vi "PCO_GetCameraDescription.vi"(8 "error in (no error)":errorcluster {"code" format="%x"}, 11 "ph":u64) -> (0 "error out":errorcluster {"code" format="%x"}, 1 "strDescription":T1 {"wSensorTypeDESC" format="%x"; "wSensorSubTypeDESC" format="%x"; "wColorPatternDESC" format="%x"; "wPatternTypeDESC" format="%x"; "dwGeneralCapsDESC1" format="%x"; "dwGeneralCapsDESC2" format="%x"; "dwGeneralCapsDESC3" format="%x"; "dwGeneralCapsDESC4" format="%x"}, 2 "ErrorMessage":i32 format="%x", 3 "ph out":u64)   [LabVIEW 2020, in "SDK.lvlib" / "CameraDescription.lvlib"]
doc: "<b>Description:</b>\nSensor and camera specific description is queried. In the returned PCO_Description structure margins for all sensor related settings and bitfields for available options of the camera are given.\n\n<b>Supported camera type:</b>\nAll cameras\n\n<b>Descriptor dependency:</b>\nNone"
uses:
  CameraDescription.lvlib
  Structures/Structures.lvlib
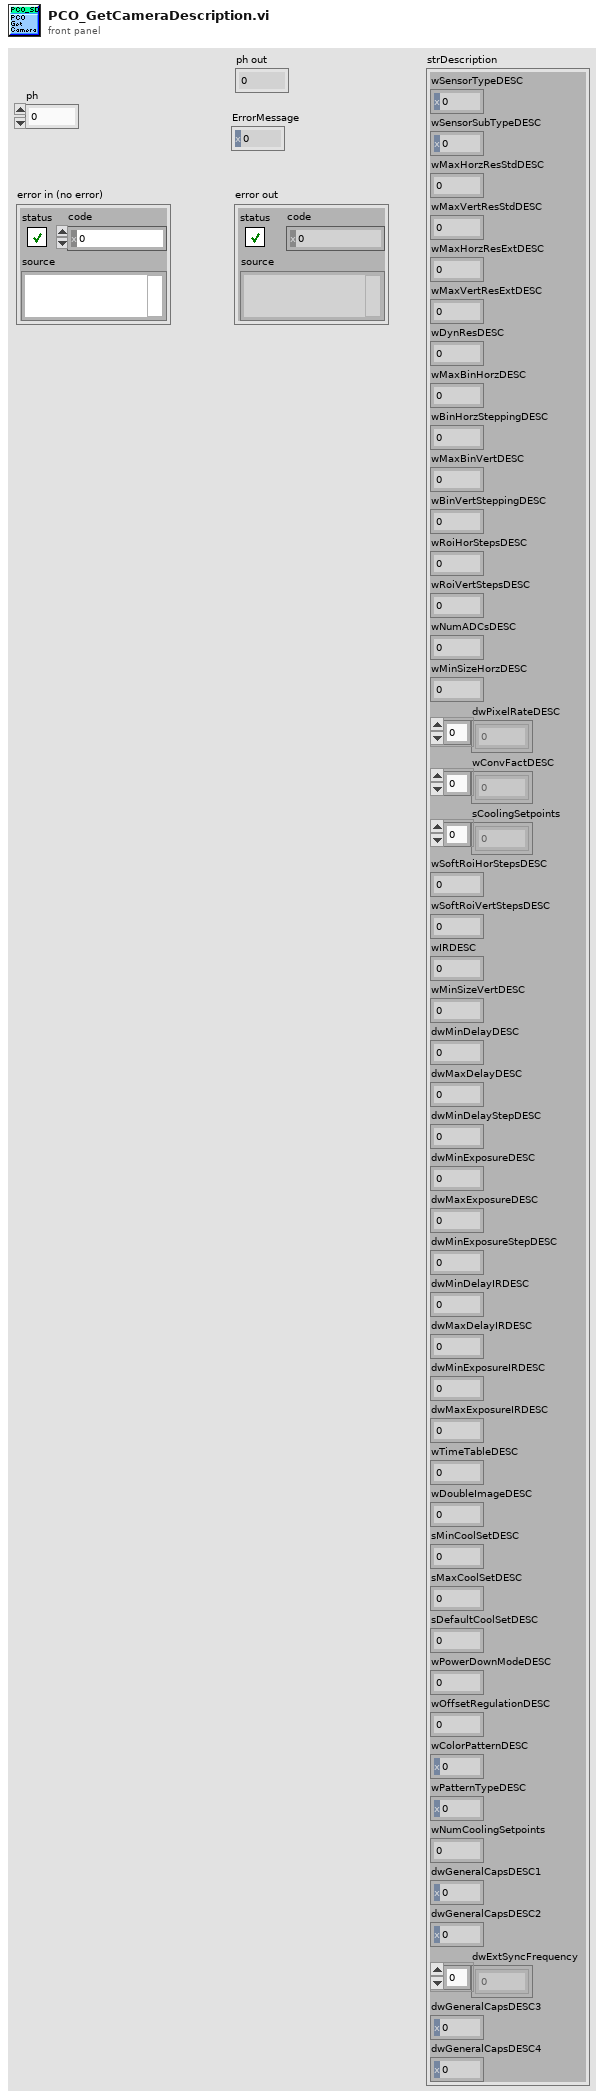
[diagram p1: front panel]
types:
  T1 = cluster{"wSensorTypeDESC":u16, "wSensorSubTypeDESC":u16, "wMaxHorzResStdDESC":u16, "wMaxVertResStdDESC":u16, "wMaxHorzResExtDESC":u16, "wMaxVertResExtDESC":u16, "wDynResDESC":u16, "wMaxBinHorzDESC":u16, "wBinHorzSteppingDESC":u16, "wMaxBinVertDESC":u16, "wBinVertSteppingDESC":u16, "wRoiHorStepsDESC":u16, "wRoiVertStepsDESC":u16, "wNumADCsDESC":u16, "wMinSizeHorzDESC":u16, "dwPixelRateDESC":u32[], "wConvFactDESC":u16[], "sCoolingSetpoints":i16[], "wSoftRoiHorStepsDESC":u16, "wSoftRoiVertStepsDESC":u16, "wIRDESC":u16, "wMinSizeVertDESC":u16, "dwMinDelayDESC":u32, "dwMaxDelayDESC":u32, "dwMinDelayStepDESC":u32, "dwMinExposureDESC":u32, "dwMaxExposureDESC":u32, "dwMinExposureStepDESC":u32, "dwMinDelayIRDESC":u32, "dwMaxDelayIRDESC":u32, "dwMinExposureIRDESC":u32, "dwMaxExposureIRDESC":u32, "wTimeTableDESC":u16, "wDoubleImageDESC":u16, "sMinCoolSetDESC":i16, "sMaxCoolSetDESC":i16, "sDefaultCoolSetDESC":i16, "wPowerDownModeDESC":u16, "wOffsetRegulationDESC":u16, "wColorPatternDESC":u16, "wPatternTypeDESC":u16, "wNumCoolingSetpoints":u16, "dwGeneralCapsDESC1":u32, "dwGeneralCapsDESC2":u32, "dwExtSyncFrequency":u32[], "dwGeneralCapsDESC3":u32, "dwGeneralCapsDESC4":u32}
  T2 = cluster{"wSize":u16, "wSensorTypeDESC":u16, "wSensorSubTypeDESC":u16, "wMaxHorzResStdDESC":u16, "wMaxVertResStdDESC":u16, "wMaxHorzResExtDESC":u16, "wMaxVertResExtDESC":u16, "wDynResDESC":u16, "wMaxBinHorzDESC":u16, "wBinHorzSteppingDESC":u16, "wMaxBinVertDESC":u16, "wBinVertSteppingDESC":u16, "wRoiHorStepsDESC":u16, "wRoiVertStepsDESC":u16, "wNumADCsDESC":u16, "wMinSizeHorzDESC":u16, "dwPixelRateDESC":cluster{u32, u32, u32, u32}, "ZZdwDummypr":cluster{u32, u32, u32, u32, u32, u32, u32, u32, u32, u32, u32, u32, u32, u32, u32, u32, u32, u32, u32, u32}, "wConvFactDESC":cluster{u16, u16, u16, u16}, "sCoolingSetpoints":cluster{i16, i16, i16, i16, i16, i16, i16, i16, i16, i16}, "ZZdwDummycv":cluster{u16, u16, u16, u16, u16, u16, u16, u16}, "wSoftRoiHorStepsDESC":u16, "wSoftRoiVertStepsDESC":u16, "wIRDESC":u16, "wMinSizeVertDESC":u16, "dwMinDelayDESC":u32, "dwMaxDelayDESC":u32, "dwMinDelayStepDESC":u32, "dwMinExposureDESC":u32, "dwMaxExposureDESC":u32, "dwMinExposureStepDESC":u32, "dwMinDelayIRDESC":u32, "dwMaxDelayIRDESC":u32, "dwMinExposureIRDESC":u32, "dwMaxExposureIRDESC":u32, "wTimeTableDESC":u16, "wDoubleImageDESC":u16, "sMinCoolSetDESC":i16, "sMaxCoolSetDESC":i16, "sDefaultCoolSetDESC":i16, "wPowerDownModeDESC":u16, "wOffsetRegulationDESC":u16, "wColorPatternDESC":u16, "wPatternTypeDESC":u16, "wDummy1":u16, "wDummy2":u16, "wNumCoolingSetpoints":u16, "dwGeneralCapsDESC1":u32, "dwGeneralCapsDESC2":u32, "dwExtSyncFrequency":cluster{u32, u32, u32, u32}, "dwGeneralCapsDESC3":u32, "dwGeneralCapsDESC4":u32, "ZZdwDummy":cluster{u32, u32, u32, u32, u32, u32, u32, u32, u32, u32, u32, u32, u32, u32, u32, u32, u32, u32, u32, u32, u32, u32, u32, u32, u32, u32, u32, u32, u32, u32, u32, u32, u32, u32, u32, u32, u32, u32, u32, u32}}
  T3 = cluster{i16, i16, i16, i16, i16, i16, i16, i16, i16, i16}
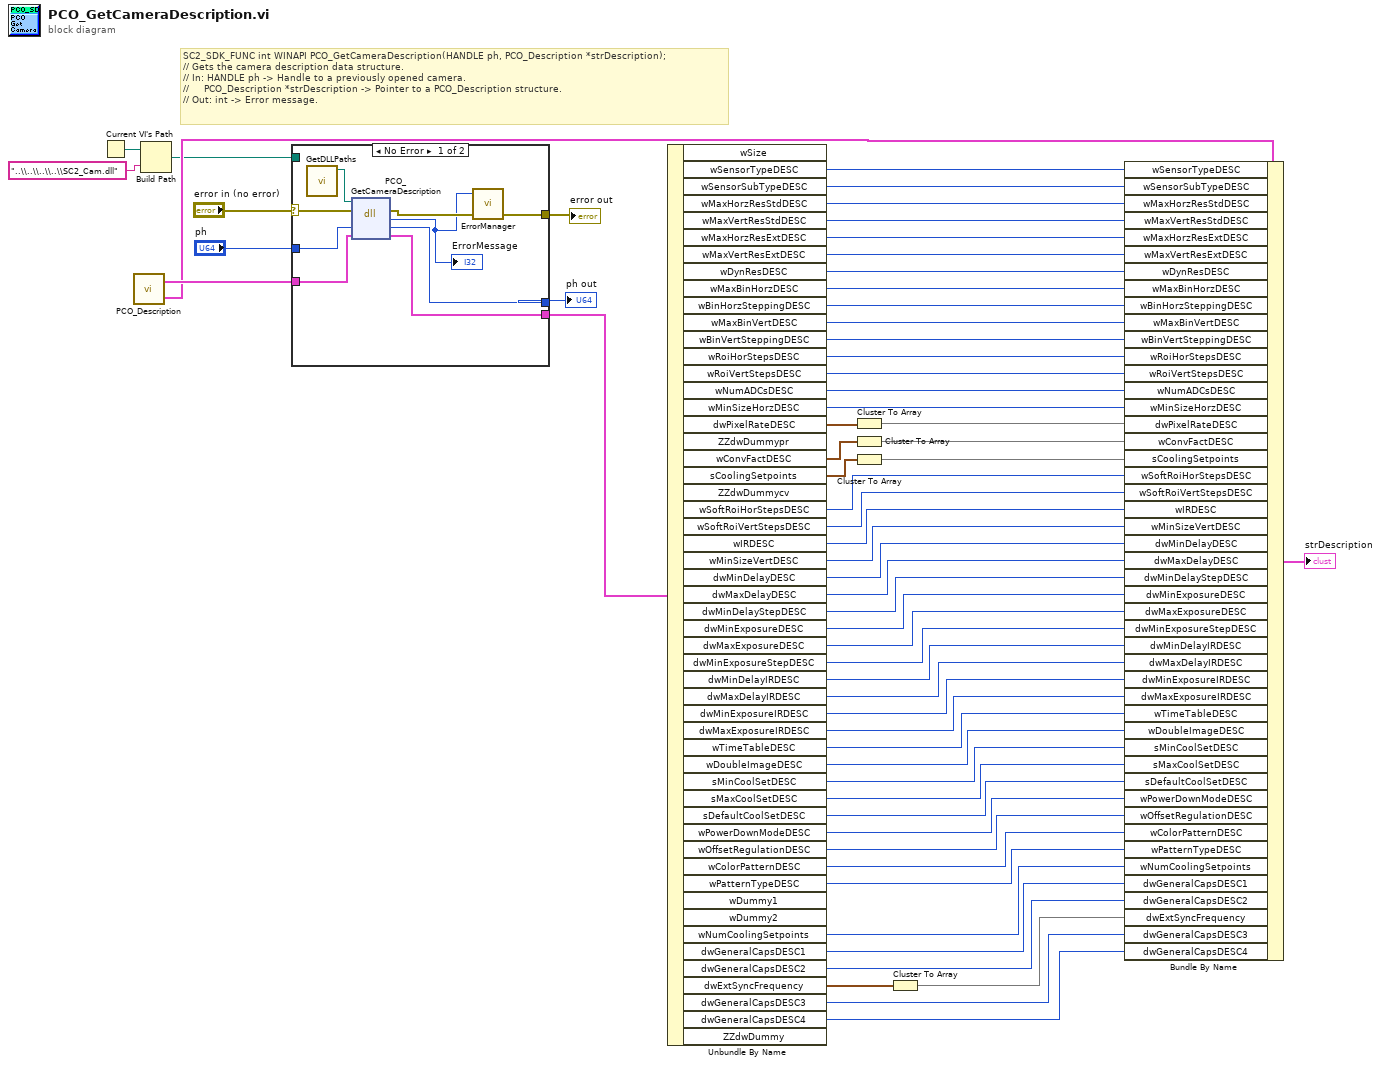
[diagram p0: block diagram]
diagram:
  # "SC2_SDK_FUNC int WINAPI PCO_GetCameraDescription(HANDLE ph, PCO_Description *strDescription);\n// Gets the camera description data structure.\n// In: HANDLE ph -> Handle to a previously opened camera.\n//     PCO_Description *strDescription -> Pointer to a PCO_Description structure.\n// Out: int -> Error message."
  n1 = Current VI's Path() -> (path=w3:path)
  n2 = call "PCO_Description.vi"() -> ("PCO_Description"=w56:T1, "PCO_Description_Raw"=w58:T2)  [unwired: 4 in, 2 out]
  n3 = Build Path(base path=w3, name or relative path="..\\..\\..\\..\\SC2_Cam.dll") -> (appended path=w2:path)
  n4 = case shown="No Error" "error in (no error)" {
    selector: "error in (no error)" -> [w64 w74]
    tunnel: "ph" -> [w71 w73]
    tunnel: [w70 w73] -> w61
    tunnel: w58 -> [w69 w72]
    tunnel: [w68 w72] -> w57
    tunnel: [w66 w74] -> w60
    tunnel: w2 -> [_ _]
    frame No Error {
      n5 = call "GetDLLPaths.vi"() -> ("SC2_Cam_Path"=w63:path)  [unwired: 9 in, 2 out]
      n6 = dll-call lib="?" fn="PCO_GetCameraDescription"(path in=w63, error in=w64, "ph"=w71, "strDescription"=w69) -> (error out=w67:errorcluster, "return type"=w65:i32, "ph"=w70:u64, "strDescription"=w68:T2)  [unwired: 1 in, 1 out]
      "ErrorMessage" <- w65
      n7 = call "ErrorManager.vi"("error in (no error)"=w67, "error code"=w65) -> ("error out"=w66:errorcluster)  [unwired: 3 in]
    }
    frame Error {
    }
  }
  "ph out" <- w61
  "error out" <- w60
  n8 = Unbundle By Name(w57) -> ("wSensorTypeDESC"=w54:u16, "wSensorSubTypeDESC"=w53:u16, "wMaxHorzResStdDESC"=w52:u16, "wMaxVertResStdDESC"=w51:u16, "wMaxHorzResExtDESC"=w50:u16, "wMaxVertResExtDESC"=w49:u16, "wDynResDESC"=w48:u16, "wMaxBinHorzDESC"=w47:u16, "wBinHorzSteppingDESC"=w46:u16, "wMaxBinVertDESC"=w45:u16, "wBinVertSteppingDESC"=w44:u16, "wRoiHorStepsDESC"=w43:u16, "wRoiVertStepsDESC"=w42:u16, "wNumADCsDESC"=w41:u16, "wMinSizeHorzDESC"=w40:u16, "dwPixelRateDESC"=w39:cluster{u32, u32, u32, u32}, "wConvFactDESC"=w37:cluster{u16, u16, u16, u16}, "sCoolingSetpoints"=w35:T3, "wSoftRoiHorStepsDESC"=w33:u16, "wSoftRoiVertStepsDESC"=w32:u16, "wIRDESC"=w31:u16, "wMinSizeVertDESC"=w30:u16, "dwMinDelayDESC"=w29:u32, "dwMaxDelayDESC"=w28:u32, "dwMinDelayStepDESC"=w27:u32, "dwMinExposureDESC"=w26:u32, "dwMaxExposureDESC"=w25:u32, "dwMinExposureStepDESC"=w24:u32, "dwMinDelayIRDESC"=w23:u32, "dwMaxDelayIRDESC"=w22:u32, "dwMinExposureIRDESC"=w21:u32, "dwMaxExposureIRDESC"=w20:u32, "wTimeTableDESC"=w19:u16, "wDoubleImageDESC"=w18:u16, "sMinCoolSetDESC"=w17:i16, "sMaxCoolSetDESC"=w16:i16, "sDefaultCoolSetDESC"=w15:i16, "wPowerDownModeDESC"=w14:u16, "wOffsetRegulationDESC"=w13:u16, "wColorPatternDESC"=w12:u16, "wPatternTypeDESC"=w11:u16, "wNumCoolingSetpoints"=w10:u16, "dwGeneralCapsDESC1"=w9:u32, "dwGeneralCapsDESC2"=w8:u32, "dwExtSyncFrequency"=w7:cluster{u32, u32, u32, u32}, "dwGeneralCapsDESC3"=w5:u32, "dwGeneralCapsDESC4"=w4:u32)  [unwired: 6 out]
  n9 = Cluster To Array(cluster=w39) -> (array=w38:u32[])
  n10 = Cluster To Array(cluster=w37) -> (array=w36:u16[])
  n11 = Cluster To Array(cluster=w35) -> (array=w34:i16[])
  n12 = Cluster To Array(cluster=w7) -> (array=w6:u32[])
  n13 = Bundle By Name(cluster=w56, "wSensorTypeDESC"=w54, "wSensorSubTypeDESC"=w53, "wMaxHorzResStdDESC"=w52, "wMaxVertResStdDESC"=w51, "wMaxHorzResExtDESC"=w50, "wMaxVertResExtDESC"=w49, "wDynResDESC"=w48, "wMaxBinHorzDESC"=w47, "wBinHorzSteppingDESC"=w46, "wMaxBinVertDESC"=w45, "wBinVertSteppingDESC"=w44, "wRoiHorStepsDESC"=w43, "wRoiVertStepsDESC"=w42, "wNumADCsDESC"=w41, "wMinSizeHorzDESC"=w40, "dwPixelRateDESC"=w38, "wConvFactDESC"=w36, "sCoolingSetpoints"=w34, "wSoftRoiHorStepsDESC"=w33, "wSoftRoiVertStepsDESC"=w32, "wIRDESC"=w31, "wMinSizeVertDESC"=w30, "dwMinDelayDESC"=w29, "dwMaxDelayDESC"=w28, "dwMinDelayStepDESC"=w27, "dwMinExposureDESC"=w26, "dwMaxExposureDESC"=w25, "dwMinExposureStepDESC"=w24, "dwMinDelayIRDESC"=w23, "dwMaxDelayIRDESC"=w22, "dwMinExposureIRDESC"=w21, "dwMaxExposureIRDESC"=w20, "wTimeTableDESC"=w19, "wDoubleImageDESC"=w18, "sMinCoolSetDESC"=w17, "sMaxCoolSetDESC"=w16, "sDefaultCoolSetDESC"=w15, "wPowerDownModeDESC"=w14, "wOffsetRegulationDESC"=w13, "wColorPatternDESC"=w12, "wPatternTypeDESC"=w11, "wNumCoolingSetpoints"=w10, "dwGeneralCapsDESC1"=w9, "dwGeneralCapsDESC2"=w8, "dwExtSyncFrequency"=w6, "dwGeneralCapsDESC3"=w5, "dwGeneralCapsDESC4"=w4) -> (→"strDescription":T1)
